vi "PXI-Update DO.vi"(0 "DO Tasks":T2[](array[typedef]), 7 "DO Waveforms":bool[][](array[boolean]), 11 "error in (no error)":errorcluster, 12 "DAQ Write State":T1) -> (15 "error out":errorcluster)   [LabVIEW 2020]
uses:
  Type Defs/Task Struct.ctl
  Type Defs/DAQ Write State enum.ctl
  Type Defs/PXI-DO Signal Bank Action.ctl
  PXI Globals.vi
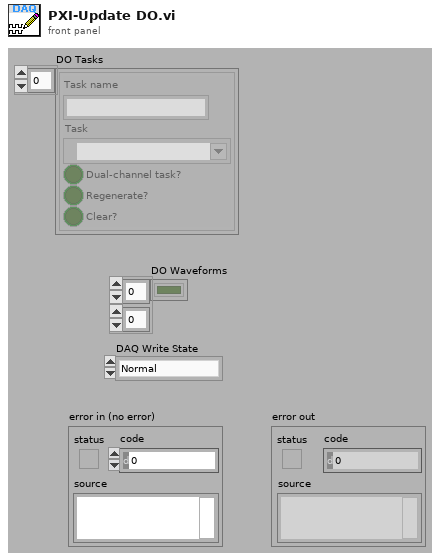
[diagram p1: front panel]
types:
  T1 = typedef "DAQ Write State enum.ctl" = enum16{"Normal", "Ramp down", "Zero buffers", "Done"}
  T2 = typedef "Task Struct.ctl" = cluster{"Task name":string, "Task":refnum<k21>, "Dual-channel task?":bool, "Regenerate?":bool, "Clear?":bool}
  T3 = typedef "PXI-DO Signal Bank Action.ctl" = enum16{"Clear", "Write", "Read"}
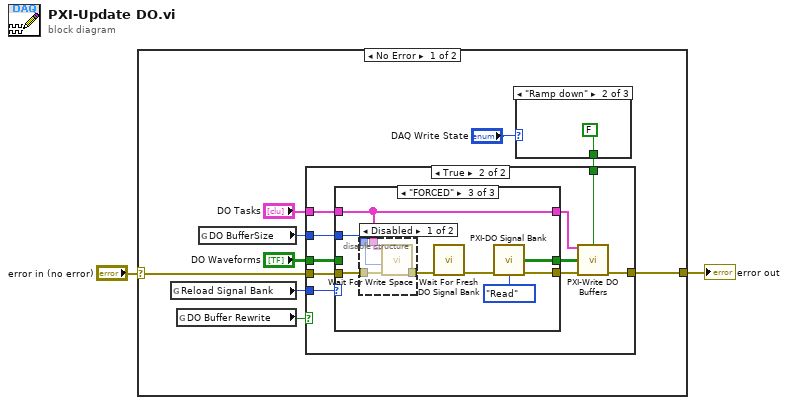
[diagram p0: block diagram]
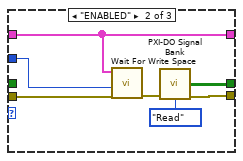
[diagram p4: hidden frame]
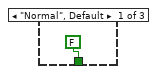
[diagram p6: hidden frame]
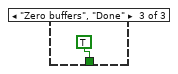
[diagram p7: hidden frame]
diagram:
  n1 = case shown="No Error" "error in (no error)" {
    selector: "error in (no error)" -> [w6 w49]
    tunnel: [w10 w49] -> w2
    frame No Error {
      n2 = global read "PXI Globals.vi" "Reload Signal Bank"() -> (w4:enum32{"OFF", "ENABLED", "FORCED"})
      n3 = global read "PXI Globals.vi" "DO Buffer Rewrite"() -> (w11:bool)
      n4 = global read "PXI Globals.vi" "DO BufferSize"() -> (w3:i32)
      n5 = case shown="\"Ramp down\"" "DAQ Write State" {
        tunnel: [FALSE FALSE TRUE] -> w8
        frame "Normal", Default {
        }
        frame "Ramp down" {
        }
        frame "Zero buffers", "Done" {
        }
      }
      n6 = case shown="True" w11 {
        tunnel: "DO Tasks" -> [_ w14]
        tunnel: w6 -> [w12 w20]
        tunnel: [w12 w22] -> w10
        tunnel: "DO Waveforms" -> [_ w17]
        tunnel: w8 -> [_ w19]
        tunnel: w4 -> [_ w16]
        tunnel: w3 -> [_ w15]
        frame False {
        }
        frame True {
          n7 = case shown="\"FORCED\"" w16 {
            tunnel: w20 -> [w25 w29 w35]
            tunnel: [w25 w32 w38] -> w21
            tunnel: [w24 w31 w39] -> w18
            tunnel: w17 -> [w24 _ _]
            tunnel: w15 -> [_ w27 w36]
            tunnel: [w23 w26 w37] -> w13
            tunnel: w14 -> [w23 w26 w37]
            frame "OFF", Default {
            }
            frame "ENABLED" {
              n8 = call "Wait For Write Space.vi"("error in (no error)"=w29, "BufferSize"=w27, "AO Tasks"=w26) -> ("error out"=w28:errorcluster)  [unwired: 6 in, 2 out]
              n9 = call "PXI-DO Signal Bank.vi"("error in (no error)"=w28, "Action"=PXI-DO_Signal_Bank_Action."Read") -> ("Array out"=w31:bool[][], "error out"=w32:errorcluster)  [unwired: 12 in]
            }
            frame "FORCED" {
              n10 = disable-structure shown="Disabled" {
                disable-tunnel: w37 -> [w44 _]
                disable-tunnel: w36 -> [w43 _]
                disable-tunnel: w35 -> [w42 w45]
                disable-tunnel: [w41 w45] -> w34
                frame Disabled {
                  n11 = call "Wait For Write Space.vi"("error in (no error)"=w42, "BufferSize"=w43, "AO Tasks"=w44) -> ("error out"=w41:errorcluster)  [unwired: 6 in, 2 out]
                }
                frame Enabled {
                }
              }
              n12 = call "Wait For Fresh DO Signal Bank.vi"("error in (no error)"=w34) -> ("error out"=w33:errorcluster)  [unwired: 10 in]
              n13 = call "PXI-DO Signal Bank.vi"("error in (no error)"=w33, "Action"=PXI-DO_Signal_Bank_Action."Read") -> ("Array out"=w39:bool[][], "error out"=w38:errorcluster)  [unwired: 12 in]
            }
          }
          n14 = call "PXI-Write DO Buffers.vi"("DO Tasks"=w13, "zero output"=w19, "DO Waveforms"=w18, "error in (no error)"=w21) -> ("error out"=w22:errorcluster)  [unwired: 10 in, 1 out]
        }
      }
    }
    frame Error {
    }
  }
  "error out" <- w2
